vi "main.vi"() -> ()   [LabVIEW 2014]
doc: "Replays a chess game using PGN game file from chess.com."
uses:
  code/board/board_actions.ctl
panel:
  out "move":string
  in  "pause":bool
  in  "prev":bool
  in  "next":bool
  in  "play":bool
  in  "reset":bool
  in  "stop":bool
  out "board":picture[][](array[picture])
  in  "board actions (reset)":T1=enum."reset"
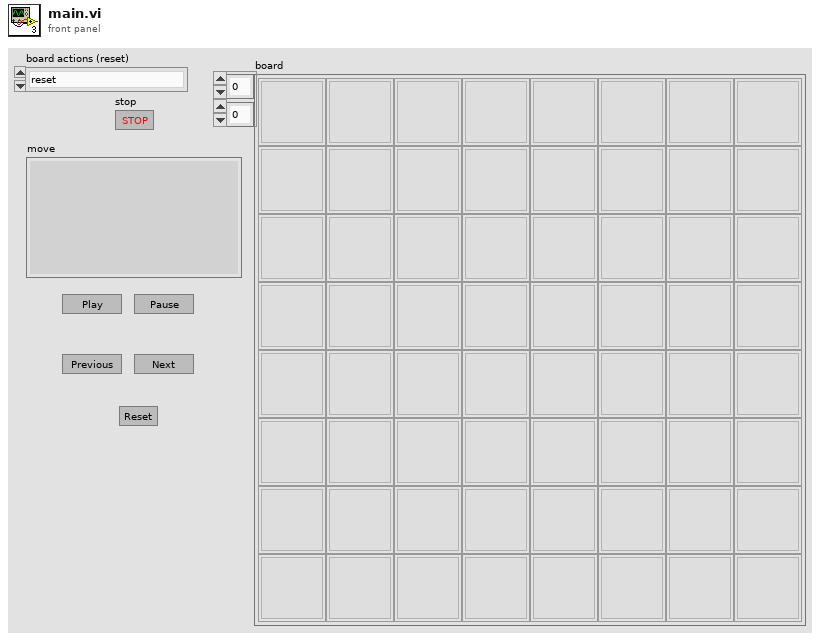
[diagram p1: front panel]
types:
  T1 = typedef "board_actions.ctl" = enum16{"move", "reset"}
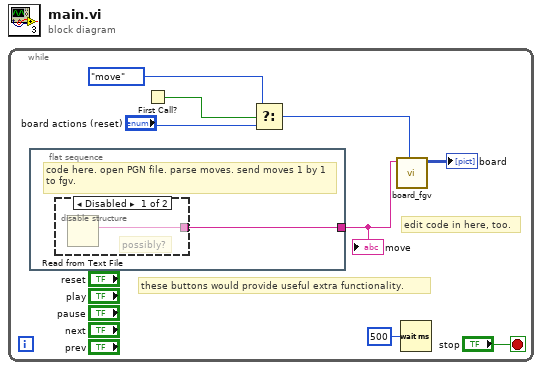
[diagram p0: block diagram]
diagram:
  n1 = while {
    stop <- "stop" stop-if-true
    # "these buttons would provide useful extra functionality."
    # "edit code in here, too."
    n2 = flat-sequence {
      tunnel: [w9] -> w1
      frame #0 {
        # "code here. open PGN file. parse moves. send moves 1 by 1 to fgv."
        n3 = disable-structure shown="Disabled" {
          disable-tunnel: [w10 _] -> w9
          frame Disabled {
            # "possibly?"
            n4 = Read from Text File() -> (text=w10:string)  [unwired: 4 in, 3 out]
          }
          frame Enabled {
          }
        }
      }
    }
    n5 = First Call?() -> (First Call?: T/F=w8:bool)
    n6 = Select(t=board_actions."move" ("board actions (reset)"), s=w8, f="board actions (reset)") -> (s? t:f=w5:T1)
    n7 = call "board_fgv.vi"("board actions (reset)"=w5, "move"=w1) -> ("board"=→"board":picture[][])  [unwired: 9 in]
    n8 = Wait (ms)(milliseconds to wait=u32 500) -> ()  [unwired: 1 out]
    "move" <- w1
  }
